vi "OBJ_read_config_files_to_fgv.vi"(8 "error_in":errorcluster, 11 "all_config_info_in":T1={"main_ini_file"={"SQL Driver"="", "SQL Server"="", "SQL Database"="", "SQL UID"="", "User table"="", "Reference table"="", "default language"="", "SCANNER COM port"=0, "SCANNER Baud rate"=0, "SCANNER Data bits"=0, "SCANNER Pairity"=enum."None", "SCANNER Stop bits"=10, "SCANNER Flow control"=0, "SCANNER Termination char"=0, "MD-L COM port"=0, "MD-L Baud rate"=0, "MD-L Data bits"=0, "MD-L Pairity"=enum."None", "MD-L Stop bits"=10, "MD-L Flow control"=0, "MD-L Termination char"=0, "MD-R COM port"=0, "MD-R Baud rate"=0, "MD-R Data bits"=0, "MD-R Pairity"=enum."None", "MD-R Stop bits"=10, "MD-R Flow control"=0, "MD-R Termination char"=0, "logout timeout [ms]"=0}, "SQL Password"="", "queue_refnums"={"MAIN_queue"=refnum, "SCANNER_queue"=refnum, "SCANNER_login"=refnum, "MD_L_queue"=refnum, "MD_L_data"=refnum, "MD_R_queue"=refnum, "MD_R_data"=refnum, "OBJ_GUI_TIMER_queue"=refnum}} {"main_ini_file"."MD-R Flow control" items=["None"=0, "XON/XOFF"=1, "RTS/CTS"=2, "DTR/DSR"=4]; "main_ini_file"."MD-R Stop bits" items=["1.0"=10, "1.5"=15, "2.0"=20]; "main_ini_file"."MD-L Flow control" items=["None"=0, "XON/XOFF"=1, "RTS/CTS"=2, "DTR/DSR"=4]; "main_ini_file"."MD-L Stop bits" items=["1.0"=10, "1.5"=15, "2.0"=20]; "main_ini_file"."SCANNER Flow control" items=["None"=0, "XON/XOFF"=1, "RTS/CTS"=2, "DTR/DSR"=4]; "main_ini_file"."SCANNER Stop bits" items=["1.0"=10, "1.5"=15, "2.0"=20]}) -> (0 "error_out":errorcluster, 3 "all_config_info_out":T1={"main_ini_file"={"SQL Driver"="", "SQL Server"="", "SQL Database"="", "SQL UID"="", "User table"="", "Reference table"="", "default language"="", "SCANNER COM port"=0, "SCANNER Baud rate"=0, "SCANNER Data bits"=0, "SCANNER Pairity"=enum."None", "SCANNER Stop bits"=10, "SCANNER Flow control"=0, "SCANNER Termination char"=0, "MD-L COM port"=0, "MD-L Baud rate"=0, "MD-L Data bits"=0, "MD-L Pairity"=enum."None", "MD-L Stop bits"=10, "MD-L Flow control"=0, "MD-L Termination char"=0, "MD-R COM port"=0, "MD-R Baud rate"=0, "MD-R Data bits"=0, "MD-R Pairity"=enum."None", "MD-R Stop bits"=10, "MD-R Flow control"=0, "MD-R Termination char"=0, "logout timeout [ms]"=0}, "SQL Password"="", "queue_refnums"={"MAIN_queue"=refnum, "SCANNER_queue"=refnum, "SCANNER_login"=refnum, "MD_L_queue"=refnum, "MD_L_data"=refnum, "MD_R_queue"=refnum, "MD_R_data"=refnum, "OBJ_GUI_TIMER_queue"=refnum}} {"main_ini_file"."MD-R Flow control" items=["None"=0, "XON/XOFF"=1, "RTS/CTS"=2, "DTR/DSR"=4]; "main_ini_file"."MD-R Stop bits" items=["1.0"=10, "1.5"=15, "2.0"=20]; "main_ini_file"."MD-L Flow control" items=["None"=0, "XON/XOFF"=1, "RTS/CTS"=2, "DTR/DSR"=4]; "main_ini_file"."MD-L Stop bits" items=["1.0"=10, "1.5"=15, "2.0"=20]; "main_ini_file"."SCANNER Flow control" items=["None"=0, "XON/XOFF"=1, "RTS/CTS"=2, "DTR/DSR"=4]; "main_ini_file"."SCANNER Stop bits" items=["1.0"=10, "1.5"=15, "2.0"=20]})   [LabVIEW 2020]
uses:
  typedef/OBJ_all_config_info.ctl
  typedef/OBJ_main_ini_file.ctl
  queues/typedef/OBJ_queue_refnums.ctl
  queues/typedef/OBJ_MAIN_queue_element.ctl
  MAIN/OBJ_MAIN_sequence_state.ctl
  queues/typedef/OBJ_SCANNER_queue_element.ctl
  SCANNER/OBJ_SCANNER_sequence_state.ctl
  queues/typedef/OBJ_MD_queue_element.ctl
  MEASURING_DEVICE/OBJ_MD_sequence_state.ctl
  queues/typedef/OBJ_GUI_TIMER_queue_element.ctl
  GUI_TIMER/OBJ_GUI_TIMER_sequence_state.ctl
  FGV/config_info/FGV_OBJ_config_info.ctl
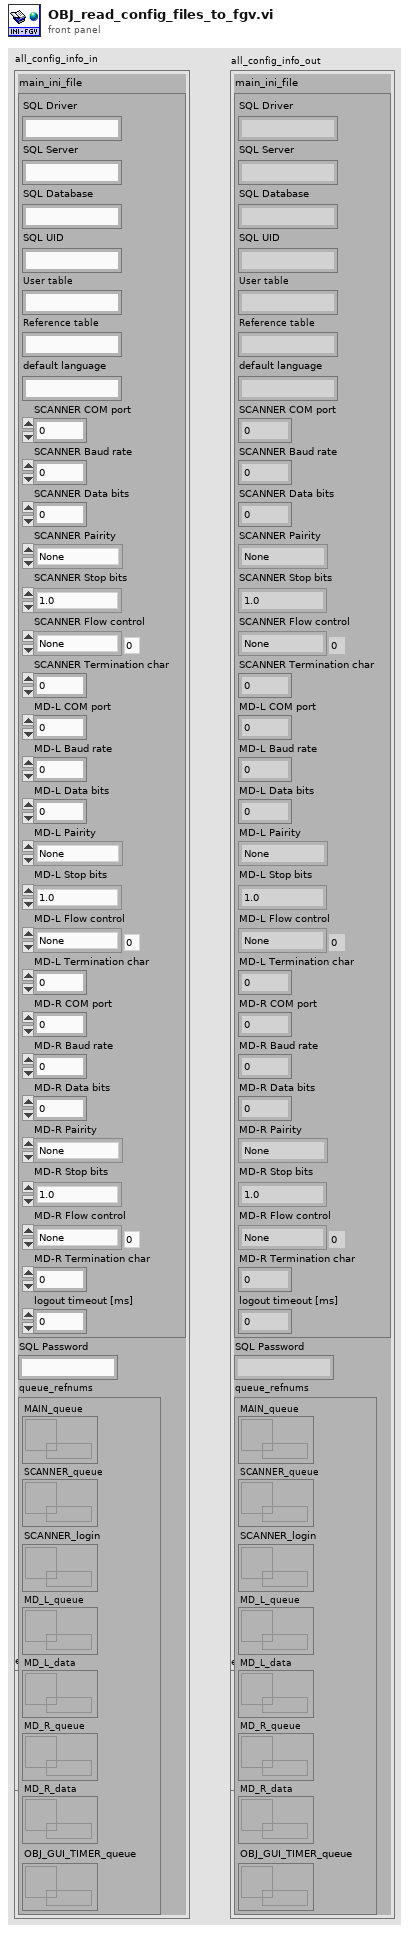
[diagram p1: front panel]
types:
  T1 = typedef "OBJ_all_config_info.ctl" = cluster{"main_ini_file":T2, "SQL Password":string, "queue_refnums":T3}
  T2 = typedef "OBJ_main_ini_file.ctl" = cluster{"SQL Driver":string, "SQL Server":string, "SQL Database":string, "SQL UID":string, "User table":string, "Reference table":string, "default language":string, "SCANNER COM port":u16, "SCANNER Baud rate":u32, "SCANNER Data bits":u16, "SCANNER Pairity":enum16{"None", "Odd", "Even", "Mark", "Space"}, "SCANNER Stop bits":u16, "SCANNER Flow control":u16, "SCANNER Termination char":u8, "MD-L COM port":u16, "MD-L Baud rate":u32, "MD-L Data bits":u16, "MD-L Pairity":enum16{"None", "Odd", "Even", "Mark", "Space"}, "MD-L Stop bits":u16, "MD-L Flow control":u16, "MD-L Termination char":u8, "MD-R COM port":u16, "MD-R Baud rate":u32, "MD-R Data bits":u16, "MD-R Pairity":enum16{"None", "Odd", "Even", "Mark", "Space"}, "MD-R Stop bits":u16, "MD-R Flow control":u16, "MD-R Termination char":u8, "logout timeout [ms]":i32}
  T3 = typedef "OBJ_queue_refnums.ctl" = cluster{"MAIN_queue":refnum<queue>, "SCANNER_queue":refnum<queue>, "SCANNER_login":refnum<queue>, "MD_L_queue":refnum<queue>, "MD_L_data":refnum<queue>, "MD_R_queue":refnum<queue>, "MD_R_data":refnum<queue>, "OBJ_GUI_TIMER_queue":refnum<queue>}
  T4 = typedef "FGV_OBJ_config_info.ctl" = enum16{"initialize", "set", "get"}
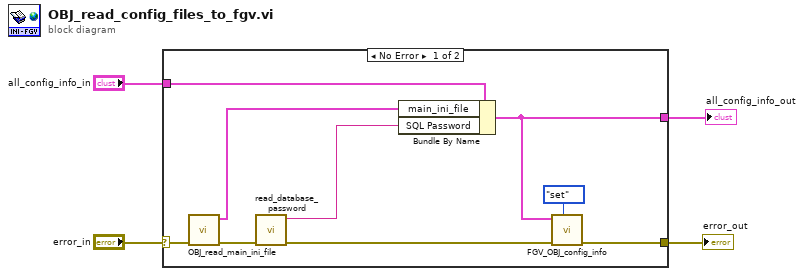
[diagram p0: block diagram]
diagram:
  n1 = case shown="No Error" "error_in" {
    selector: "error_in" -> [w13 w15]
    tunnel: [w11 w15] -> w4
    tunnel: [w5 w14] -> w1
    tunnel: "all_config_info_in" -> [w10 w14]
    frame No Error {
      n2 = call "OBJ_read_main_ini_file.vi"("error_in"=w13) -> ("error_out"=w9:errorcluster, "main_ini_file_out"=w6:T2)  [unwired: 7 in, 2 out]
      n3 = call "read_database_password.vi"("error_in"=w9) -> ("error_out"=w8:errorcluster, "database_password"=w7:string)  [unwired: 8 in]
      n4 = Bundle By Name(cluster=w10, "main_ini_file"=w6, "SQL Password"=w7) -> (w5:T1)
      n5 = call "FGV_OBJ_config_info.vi"("options"=FGV_OBJ_config_info."set", "error_in"=w8, "all_config_info_in"=w5) -> ("error_out"=w11:errorcluster)  [unwired: 7 in, 1 out]
    }
    frame Error {
    }
  }
  "error_out" <- w4
  "all_config_info_out" <- w1
